vi "TEST_L0_SUMnADDS_NEW.vi"(7 "Serial number":string="SN018", 8 "error in":errorcluster, 11 "Instrument VISA in":T1={"AWG VISA"="generadorpulsos", "Oscilloscope  VISA "="Oscilloscope", "Integration Board IP"="172.16.7.43", "connection ID"=refnum, "report out"=refnum, "report file path"=path "C:/Documents and Settings/CTA_LAB01/Desktop/L0_Asic/L0 Asic Test Data"}) -> (0 "error out":errorcluster={"status"=TRUE, "code"=-1073807343, "source"="VISA Open in Agilent 81150.lvlib:Initialize.vi->Set_Gen_Conf.vi->L0_Sum_Adder.vi"}, 3 "Instrument VISA out":T1={"AWG VISA"="generadorpulsos", "Oscilloscope  VISA "="Oscilloscope", "Integration Board IP"="172.16.7.43", "connection ID"=refnum, "report out"=refnum, "report file path"=path "C:/Documents and Settings/CTA_LAB01/Desktop/L0_Asic/L0 Asic Test Data"})   [LabVIEW 2009]
uses:
  <vilib>/Utility/NIReport.llb/NI_report.lvclass
  <vilib>/Utility/NIReport.llb/HTML/NI_HTML.lvclass
  Sum_Abrilader/L0_Sum_Adder Folder/C/Program Files/National Instruments/LabVIEW 2012/instr.lib/Agilent 8000 Series/Public/Configure/Configure Math (Binary Operation).vi
  <vilib>/Utility/file.llb/Write To Spreadsheet File (string).vi
  Sum_Abrilader/L0_Sum_Adder Folder/C/Program Files/National Instruments/LabVIEW 2012/instr.lib/Agilent 8000 Series/Public/Data/Low Level/Fetch Measurement (More).vi
  Sum_Abrilader/L0_Sum_Adder Folder/C/Program Files/National Instruments/LabVIEW 2012/instr.lib/Agilent 8000 Series/Agilent 8000 Series.lvlib
panel:
  in  "Channels Combinations":i32[](array[numeric])=[3, 12, 48, 96, 7, 28, 112, 15, 120, 31, 124, 63, 126, 127]
  in  "Voltage Array":dbl[](array[numeric])=[0.05, 0.2]
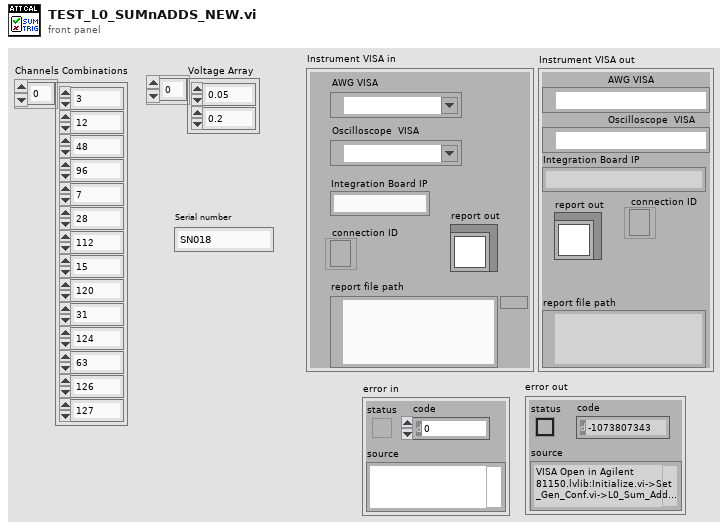
[diagram p1: front panel]
types:
  T1 = cluster{"AWG VISA":refnum<visa-resource-name>, "Oscilloscope  VISA ":refnum<visa-resource-name>, "Integration Board IP":string, "connection ID":refnum<k5>, "report out":refnum<class "NI_report.lvclass">, "report file path":path}
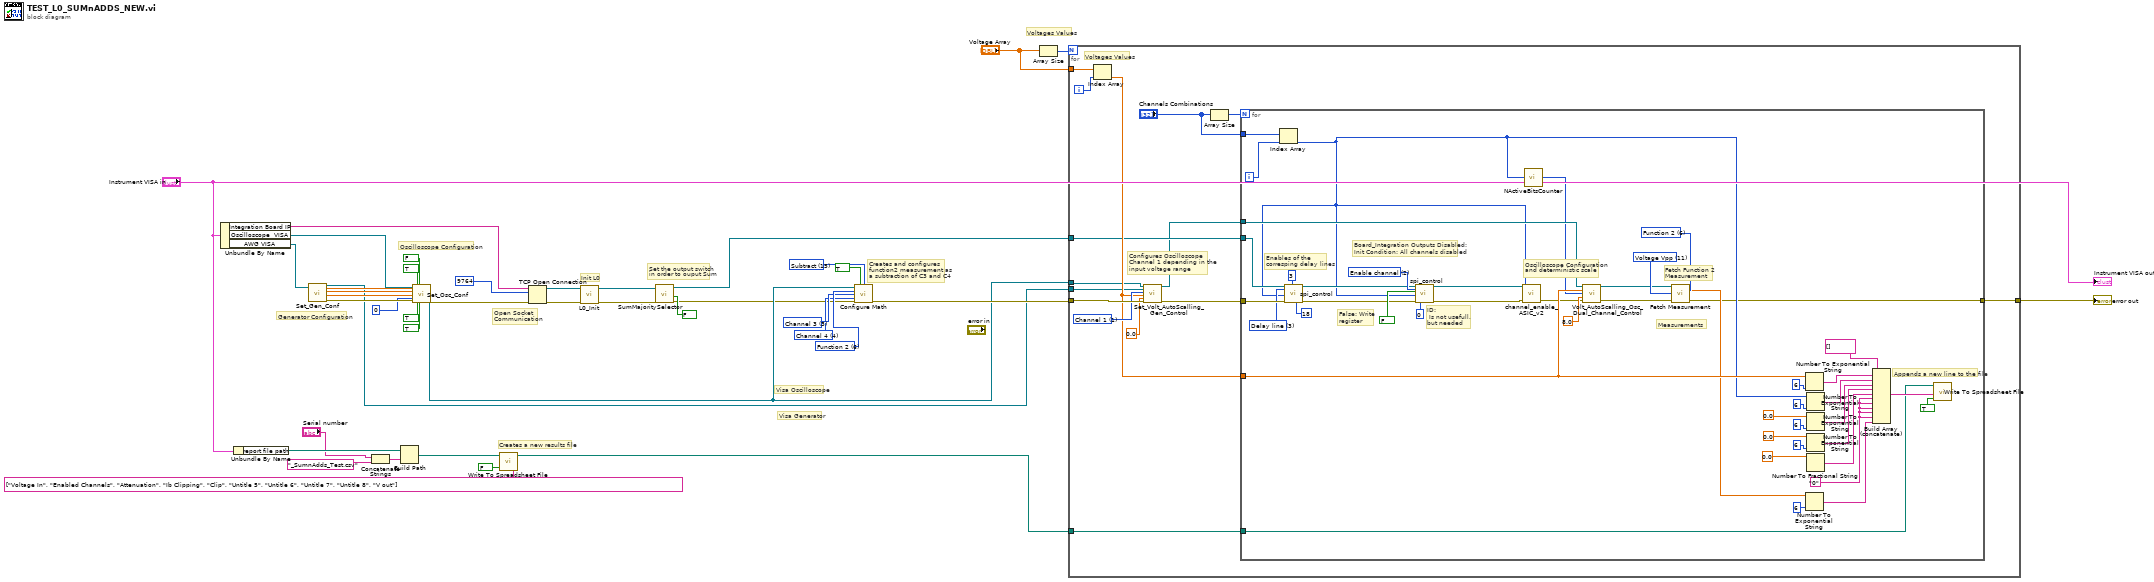
[diagram p0: block diagram]
diagram:
  w28 = u16 6 items=["Function 1"=5, "Function 2"=6, "Function 3"=7, "Function 4"=8] ("Math Channel (5: Function 1)")
  w29 = u16 15 items=["Add"=12, "Divide"=13, "Multiply"=14, "Subtract"=15, "Common Mode"=16, "Versus"=17] ("Math Operation (12: Add)")
  w27 = 3 items=["Channel 1"=1, "Channel 2"=2, "Channel 3"=3, "Channel 4"=4] ("Channel (1: Channel 1)")
  w26 = 4 items=["Channel 1"=1, "Channel 2"=2, "Channel 3"=3, "Channel 4"=4] ("Channel (1: Channel 1)")
  # "Init L0"
  # "Creates and configures\nfunction2 measurement as\na subtraction of C3 and C4"
  # "Creates a new results file"
  # "Set the output switch\nin order to ouput Sum"
  # "Open Socket\nCommunication"
  # "Visa Generator"
  # "Visa Oscilloscope"
  # "Oscilloscope Configuration"
  # "Voltages Values"
  # "Generator Configuration"
  n1 = Unbundle By Name("Instrument VISA in") -> ("Integration Board IP"=w11:string, "Oscilloscope  VISA"=w12:refnum<visa-resource-name>, "AWG VISA"=w13:refnum<visa-resource-name>)
  n2 = Unbundle By Name("Instrument VISA in") -> ("report file path"=w8:path)
  n3 = call "Set_Gen_Conf.vi"("AWG VISA"=w13) -> ("Amplitude 1 OUT"=w36:dbl, "VISA resource name out"=w21:refnum<visa-resource-name>, "Pulse Width in seconds 1 OUT"=w35:dbl, "Trigger Level 1"=w34:dbl, "error out"=w33:errorcluster)  [unwired: 11 in, 3 out]
  n4 = Concatenate Strings("Serial number", "_SumnAdds_Test.csv" ("format string")) -> (w9:string)
  n5 = Build Path(base path=w8, name or relative path=w9) -> (appended path=w6:path)
  n6 = call "Set_Osc_Conf.vi"("VISA resource name"=w12, "Amplitude IN"=w36, "Trigger Level IN"=w34, "Pulse Width in seconds IN"=w35, "Position 1"=0, "error in (no error)"=w33, "Channel 1"=TRUE, "Channel 3"=TRUE, "Channel 2"=FALSE, "Channel 4"=TRUE) -> ("VISA resource name out"=w20:refnum<visa-resource-name>, "error out"=w19:errorcluster)  [unwired: 8 in]
  n7 = call-poly <vilib>:"Write To Spreadsheet File.vi"("append to file? (new file:F)"=FALSE, "1D data"=string[] ["Voltage In", "Enabled Channels", "Attenuation", "Ib Clipping", "Clip", "Untitle 5", "Untitle 6", "Untitle 7", "Untitle 8", "V out"], "file path (dialog if empty)"=w6) -> ("new file path (Not A Path if cancelled)"=w22:path)  [unwired: 5 in]
  n8 = TCP Open Connection(address=w11, remote port or service name=u16 9764, error in (no error)=w19) -> (connection ID=w4:refnum<k5>, error out=w3:errorcluster)  [unwired: 2 in]
  n9 = call "L0_Init.vi"("error in"=w3, "connection ID in"=w4) -> ("error out"=w1:errorcluster, "connection ID out"=w2:refnum<k5>)  [unwired: 8 in]
  n10 = call "SumMajoritySelector.vi"("On Sum\nOff Majority"=FALSE ("On Sum\nOff Majority"), "error in (no error)"=w1, "connection ID"=w2) -> ("error out"=w16:errorcluster, "connection ID out"=w17:refnum<k5>)  [unwired: 5 in]
  n11 = call-poly "Configure Math.vi"("VISA resource name"=w20, "Enable Math Channel (T:Enable)"=TRUE, "Math Operation (12: Add)"=w29, "Math Channel (5: Function 1)"=w28, "Math Operand (1: Channel 1)"=w27, "Math Operand (2: Channel 2)"=w26, "error in (no error)"=w16) -> ("error out"=w25:errorcluster)  [unwired: 7 in, 1 out]
  n12 = Array Size(array="Voltage Array") -> (size(s)=w32:i32)
  n13 = for {
    N: w32 -> [_]
    tunnel: w17 -> [w47]
    tunnel: w25 -> [w54]
    tunnel: "Voltage Array" -> [w56]
    tunnel: w22 -> [w51]
    tunnel: w21 -> [w49]
    tunnel: w20 -> [w48]
    tunnel: [w42] -> w14
    i -> [w55]
    w53 = 1 items=["Channel 1"=1, "Channel 2"=2, "Channel 3"=3, "Channel 4"=4] ("Channel")
    # "Configures Oscilloscope\nChannel 1 depending in the \ninput voltage range"
    # "Voltages Values"
    n14 = Index Array(array=w56, index=w55) -> (element=w52:dbl)
    n15 = call "Set_Volt_AutoScalling_Gen_Control.vi"("VISA Oscilloscope"=w48, "VISA Generator"=w49, "Channel"=w53, "Amplitude"=w52, "DC Offset"=0.0, "error in (no error)"=w54) -> ("VISA Oscilloscope"=w45:refnum<visa-resource-name>, "error out"=w46:errorcluster)  [unwired: 11 in, 1 out]
    n16 = Array Size(array="Channels Combinations") -> (size(s)=w44:i32)
    n17 = for {
      N: w44 -> [_]
      tunnel: w47 -> [w75]
      tunnel: w52 -> [w83]
      tunnel: w51 -> [w84]
      tunnel: w46 -> [w74]
      tunnel: w45 -> [w62]
      tunnel: "Channels Combinations" -> [w60]
      tunnel: [w57] -> w42
      i -> [w59]
      w68 = u16 2 items=["Attenuation", "Clipping", "Enable channel", "Delay line", "ASIC"] ("Device")
      w71 = u16 3 items=["Attenuation", "Clipping", "Enable channel", "Delay line", "ASIC"] ("Device")
      w90 = "0" ("F-format string")
      w100 = 11 items=["Rise Time", "Fall Time", "Frequency", "Period", "Voltage RMS(AC)", "Voltage RMS(DC)", "Voltage RMS (AC,cycle)", "Voltage RMS (DC,cycle)", "Voltage Max", "Voltage Min", "Voltage Middle", "Voltage Vpp", "Voltage High", "Voltage Low", "Voltage Average", "Voltage Average (cycle)", "Width Negative", "Width Positive", "Duty Cycle Positive", "Amplitude", "Overshoot", "Preshoot", "Voltage Base", "Voltage Upper", "Time Max", "Time Min", "Color Grade Crossing", "Color Grade Eye Width", "Color Grade Eye Height", "Color Grade Eye Q-Factory", "Color Grade Eye Duty Cycle Distortion(Percent)", "Color Grade Eye Duty Cycle Distortion(Time)", "Color Grade Eye Jitter(PP)", "Color Grade Eye Width(RMS)", "Cycle-cycle Duty Jitter(Rising)", "Cycle-cycle Duty Jitter(Falling)", "Cycle-cycle Jitter(Rising)", "Cycle-cycle Jitter(Falling)", "Cycle-cycle - Width", "Cycle-cycle + Width", "Date Rate", "Unit Interval", "FFT Delta Frequency", "FFT Delta Magnitude", "FFT Frequency", "FFT Magnitude", "Slew Rate", "Area (Entire Display)", "Area(Single Cycle)", "Duty Cycle (Rising)", "Duty Cycle (Falling)"] ("Measurement Function (0: Rise Time)")
      w101 = 6 items=["Channel 1"=1, "Channel 2"=2, "Channel 3"=3, "Channel 4"=4, "Function 1"=5, "Function 2"=6, "Function 3"=7, "Function 4"=8, "Memory 1"=9, "Memory 2"=10, "Memory 3"=11, "Memory 4"=12] ("Channel (1: Channel 1)")
      # "Appends a new line to the file"
      # "Fetch Function 2\nMeasurement"
      # "Enables of the\ncorresping delay lines"
      # "False: Write\nregister"
      # "ID:\n Is not usefull, \nbut needed"
      # "Board_Integration Outputs Disabled:\nInit Condition: All channels disabled"
      # "Measurements"
      # "Oscilloscope Configuration \nand deterministic scale"
      n18 = Index Array(array=w60, index=w59) -> (element=w58:i32)
      n19 = call "spi_control.vi"("connection ID"=w75, "Device"=w71, "Data"=w58, "Register or channel"=18, "error out 3"=w74, "chip delay"=3) -> ("connection ID out"=w66:refnum<k5>, "error out 2"=w65:errorcluster)  [unwired: 6 in, 6 out]
      n20 = call "spi_control.vi"("connection ID"=w66, "Device"=w68, "Read/#write"=FALSE, "Data"=w58, "error out 3"=w65, "Id in"=0) -> ("connection ID out"=w64:refnum<k5>, "error out 2"=w63:errorcluster)  [unwired: 6 in, 6 out]
      n21 = call "channel_enable_ASIC_v2.vi"("error in"=w63, "Channel Combination"=w58, "Connection ID in"=w64) -> ("error out"=w70:errorcluster)  [unwired: 7 in, 1 out]
      n22 = call "NActiveBitsCounter.vi"("Input Number"=w58) -> ("N High Bits"=w61:i32)
      n23 = call "Volt_AutoScalling_Osc_Dual_Channel_Control.vi"("VISA Oscilloscope"=w62, "Voltage In"=w83, "N Channels"=w61, "Offset Divider"=8.0, "error in"=w70) -> ("VISA resource name out"=w81:refnum<visa-resource-name>, "error out"=w79:errorcluster)  [unwired: 9 in]
      n24 = call-poly "Fetch Measurement.vi"("VISA resource name"=w81, "Channel (1: Channel 1)"=w101, "Measurement Function (0: Rise Time)"=w100, "error in (no error)"=w79) -> ("Measurement"=w80:dbl, "error out"=w57:errorcluster)  [unwired: 9 in, 1 out]
      n25 = Number To Exponential String(number=w83, precision (6)=i16 6) -> (E-format string=w91:string)  [unwired: 2 in]
      n26 = Number To Exponential String(number=w80, precision (6)=i16 6) -> (E-format string=w89:string)  [unwired: 2 in]
      n27 = Number To Exponential String(number=w58, precision (6)=i16 6) -> (E-format string=w99:string)  [unwired: 2 in]
      n28 = Number To Exponential String(number=0.0 ("Offset Divider"), precision (6)=i16 6) -> (E-format string=w98:string)  [unwired: 2 in]
      n29 = Number To Exponential String(number=0.0 ("Offset Divider"), precision (6)=i16 6) -> (E-format string=w96:string)  [unwired: 2 in]
      n30 = Number To Fractional String(number=0.0 ("Offset Divider")) -> (F-format string=w92:string)  [unwired: 3 in]
      n31 = Build Array (concatenate)(string[] [] ("array"), w91, w99, w98, w96, w92, w90, w90, w90, w90, w90, w89) -> (w85:string[])
      n32 = call-poly <vilib>:"Write To Spreadsheet File.vi"("append to file? (new file:F)"=TRUE, "1D data"=w85, "file path (dialog if empty)"=w84) -> ()  [unwired: 5 in, 1 out]
    }
  }
  "error out" <- w14
  "Instrument VISA out" <- "Instrument VISA in"
